vi "Restore Writable Controls.vi"(8 "error in (no error)":errorcluster, 11 "Settings in":refnum<class "Settings.lvclass">) -> (0 "error out":errorcluster, 3 "Settings out":refnum<class "Settings.lvclass">)   [LabVIEW 2017, in "Settings.lvclass"]
doc: "Write initial values to Writable Controls."
uses:
  Settings.lvclass
  Settings.lvclass/Settings.ctl
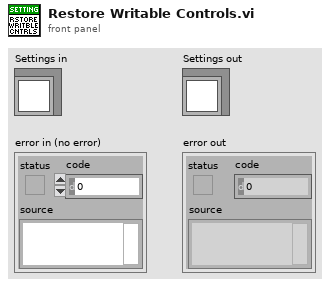
[diagram p1: front panel]
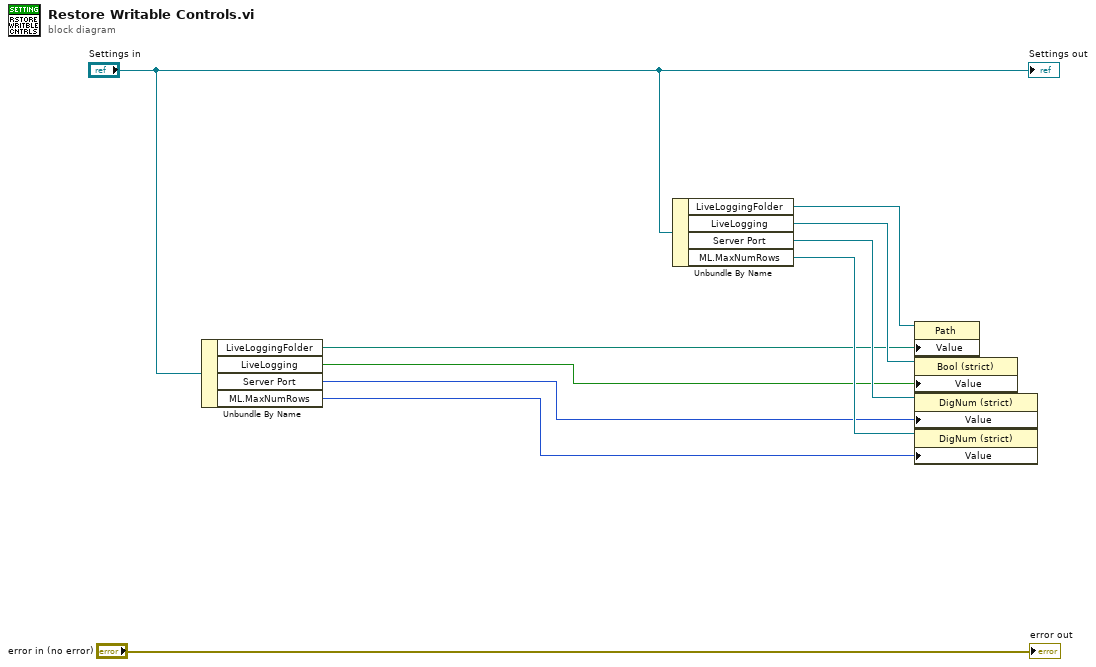
[diagram p0: block diagram]
diagram:
  n1 = Unbundle By Name("Settings in") -> ("LiveLoggingFolder"=w4:path, "LiveLogging"=w3:bool, "Server Port"=w2:u16, "ML.MaxNumRows"=w1:u16)
  n2 = Unbundle By Name("Settings in") -> ("LiveLoggingFolder"=w8:refnum<vi>, "LiveLogging"=w7:refnum<vi>, "Server Port"=w9:refnum<vi>, "ML.MaxNumRows"=w6:refnum<vi>)
  n3 = property class="Path"(reference=w8, "Value"=w4) -> ()  [unwired: 1 in, 2 out]
  n4 = property class="Bool (strict)"(reference=w7, "Value"=w3) -> ()  [unwired: 1 in, 2 out]
  n5 = property class="DigNum (strict)"(reference=w9, "Value"=w2) -> ()  [unwired: 1 in, 2 out]
  n6 = property class="DigNum (strict)"(reference=w6, "Value"=w1) -> ()  [unwired: 1 in, 2 out]
  "error out" <- "error in (no error)"
  "Settings out" <- "Settings in"
